vi "MainConvertiMisure_OUTPUT.vi"(10 "AO non scalati":T1, 11 "Caratteristiche Caricate":string[][](array[string])) -> (2 "AO scalati":T1)   [LabVIEW 2019]
uses:
  TypeDef/Lista AO sistema.ctl
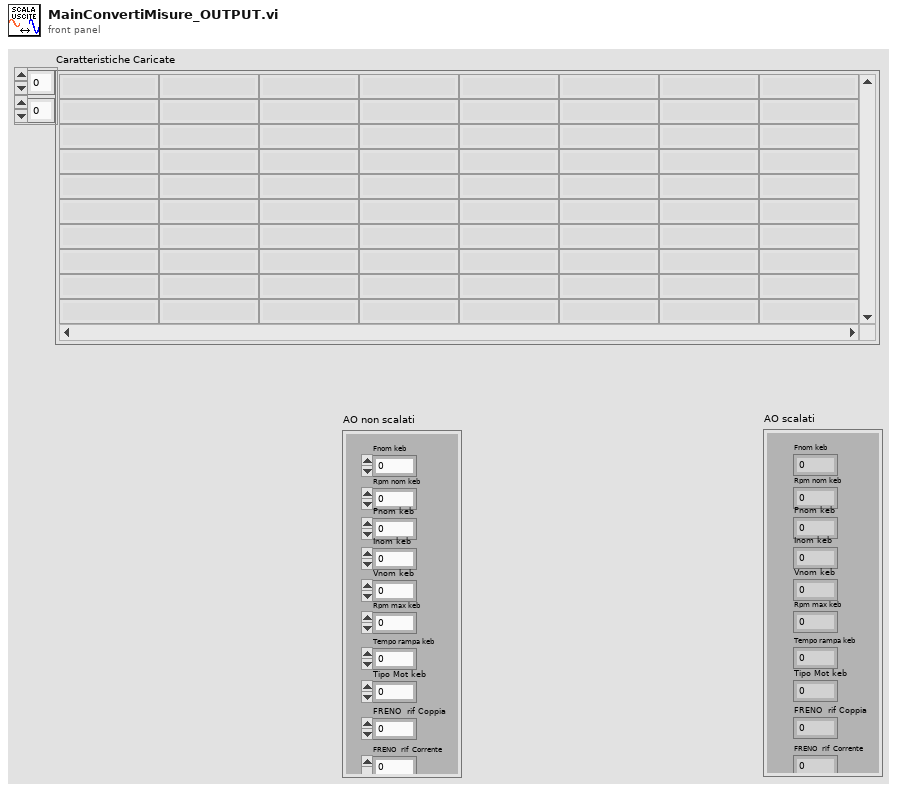
[diagram p1: front panel]
types:
  T1 = typedef "Lista AO sistema.ctl" = cluster{"FRENO1 rif vel":dbl, "FRENO1 rif Coppia":dbl, "FRENO2 rif vel":dbl, "FRENO2 rif Coppia":dbl, "ALIM1 rif V":dbl, "ALIM1 rif F":dbl, "ALIM2 rif V":dbl, "ALIM2 rif F":dbl, "ALIM3 rif V":dbl, "ALIM3 rif F":dbl, "Fnom keb":dbl, "Rpm nom keb":dbl, "Pnom keb":dbl, "Inom keb":dbl, "Vnom keb":dbl, "Rpm max keb":dbl, "Tempo rampa keb":dbl, "Tipo Mot keb":dbl, "FRENO  rif Coppia ":dbl, "FRENO  rif  Corrente":dbl}
  T2 = cluster{"[0]":dbl, "[1]":dbl, "[2]":dbl, "[3]":dbl, "[4]":dbl, "[5]":dbl, "[6]":dbl, "[7]":dbl, "[8]":dbl, "[9]":dbl, "[10]":dbl, "[11]":dbl, "[12]":dbl, "[13]":dbl, "[14]":dbl, "[15]":dbl, "[16]":dbl, "[17]":dbl, "[18]":dbl, "[19]":dbl}
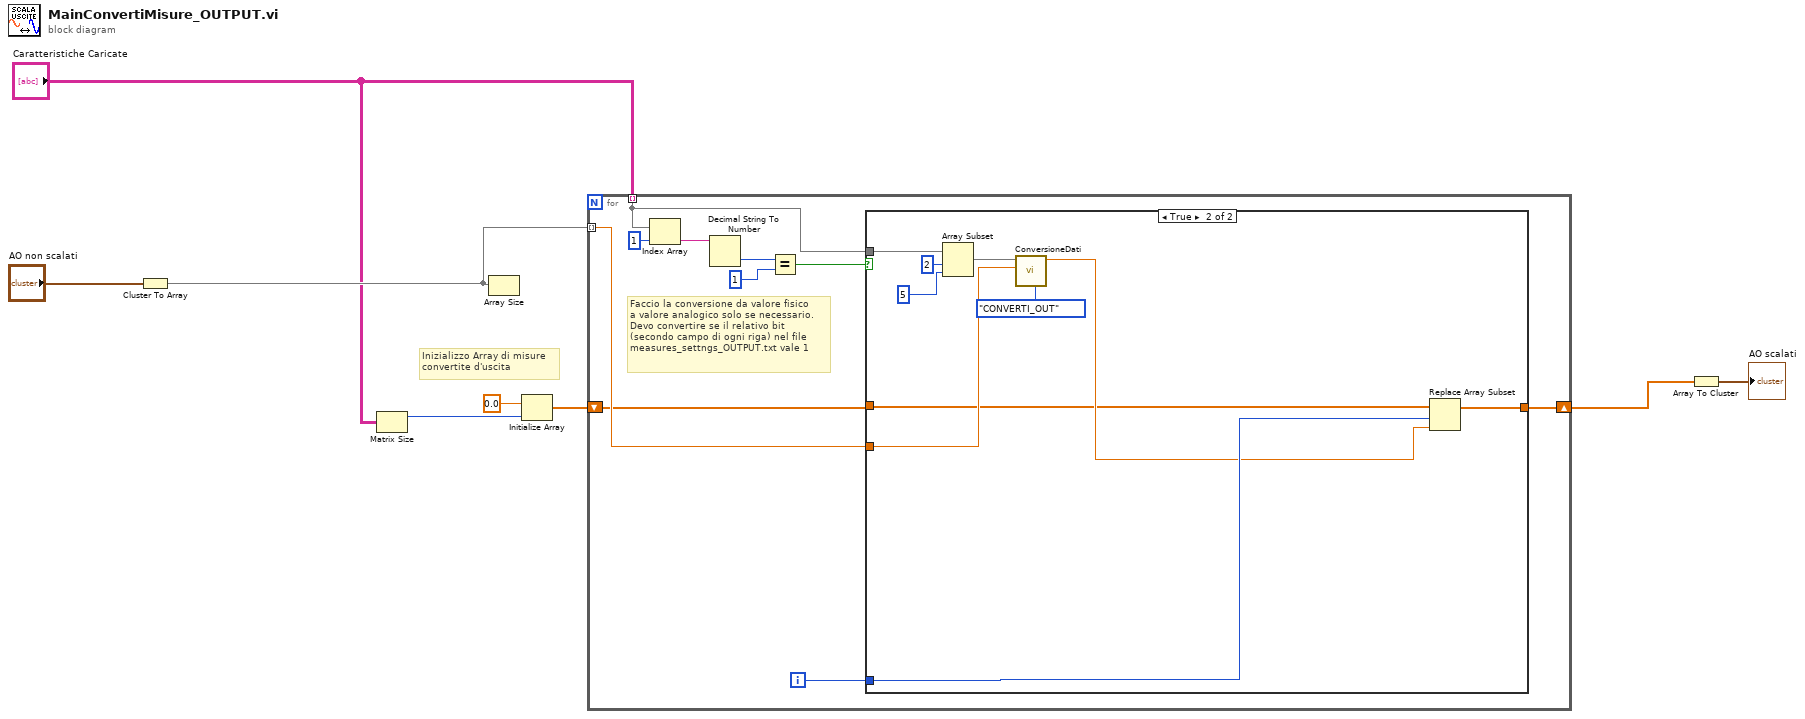
[diagram p0: block diagram]
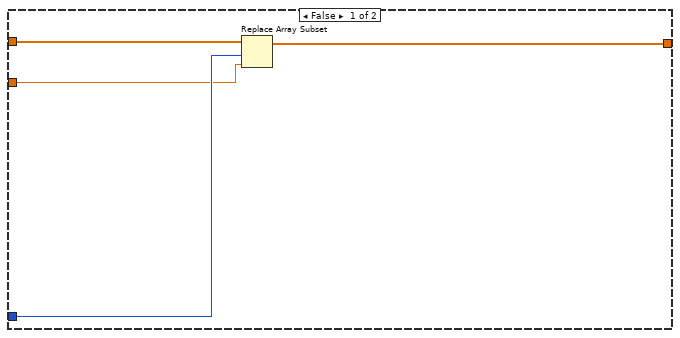
[diagram p2: hidden frame]
diagram:
  # "Inizializzo Array di misure \nconvertite d'uscita"
  n1 = Cluster To Array(cluster="AO non scalati") -> (array=w5:dbl[])
  n2 = Matrix Size(0:"Caratteristiche Caricate") -> (1:w1:i32)  [unwired: 1 out]
  n3 = Array Size(array=w5) -> ()  [unwired: 1 out]
  n4 = Initialize Array(0.0, w1) -> (w7:dbl[])
  n5 = for {
    tunnel: w5 -> [w13] mode=indexing
    tunnel: "Caratteristiche Caricate" -> [w10] mode=indexing
    shift-right: [w11] -> w4
    shift-left: w7 -> [w12]
    i -> [w9]
    # "Faccio la conversione da valore fisico\na valore analogico solo se necessario. \nDevo convertire se il relativo bit \n(secondo campo di ogni riga) nel file \nmeasures_settngs_OUTPUT.txt vale 1"
    n6 = Index Array(array=w10, index=1) -> (element=w17:string)
    n7 = Decimal String To Number(string=w17) -> (number=w16:i32)  [unwired: 2 in, 1 out]
    n8 = Equal?(x=w16, y=1) -> (x = y?=w14:bool)
    n9 = case shown="True" w14 {
      tunnel: w13 -> [w21 w28]
      tunnel: w12 -> [w19 w23]
      tunnel: w9 -> [w22 w32]
      tunnel: [w20 w31] -> w11
      tunnel: w10 -> [_ w30]
      frame False {
        n10 = Replace Array Subset(array=w19, new element=w21, index=w22) -> (w20:dbl[])
      }
      frame True {
        n11 = Array Subset(array=w30, index=2, length=5 ("index")) -> (w29:string[])
        n12 = call "ConversioneDati.vi"("Stato Conversione"=enum16{"CONVERTI_IN", "CONVERTI_OUT"}."CONVERTI_OUT", "Data"=w28, "Impostazioni Conversione"=w29) -> ("Dato Convertito"=w25:dbl)  [unwired: 8 in]
        n13 = Replace Array Subset(array=w23, new element=w25, index=w32) -> (w31:dbl[])
      }
    }
  }
  n14 = Array To Cluster(array=w4) -> (cluster=→"AO scalati":T2)
